vi "Insert Vi by Node.vi"(8 "error in":errorcluster caption="错误输入（无错误）", 9 "dynamic VI*":refnum<vi>, 10 "Node*":refnum<data-value>, 11 "PanelRootNode 输入":refnum<class "PanelRootNode.lvclass"> caption="DNL_LabVIEW Object in") -> (0 "error out":errorcluster caption="错误输出", 3 "PanelRootNode 输出":refnum<class "PanelRootNode.lvclass"> caption="DNL_LabVIEW Object out")   [LabVIEW 2013, in "PanelRootNode.lvclass"]
uses:
  PanelRootNode.lvclass
  PanelObject/PanelObject.lvclass
  PanelLinkNode/PanelLinkNode.lvclass/PanelLinkNode.ctl
  PanelDataNode/PanelDataNode.lvclass
  PanelLinkNode/PanelLinkNode.lvclass
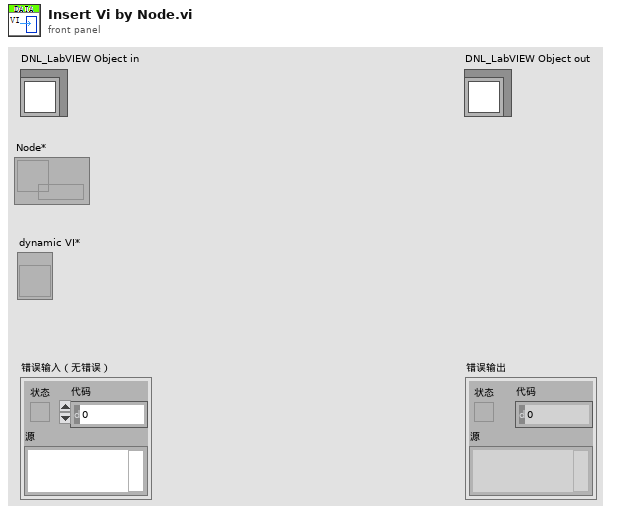
[diagram p1: front panel]
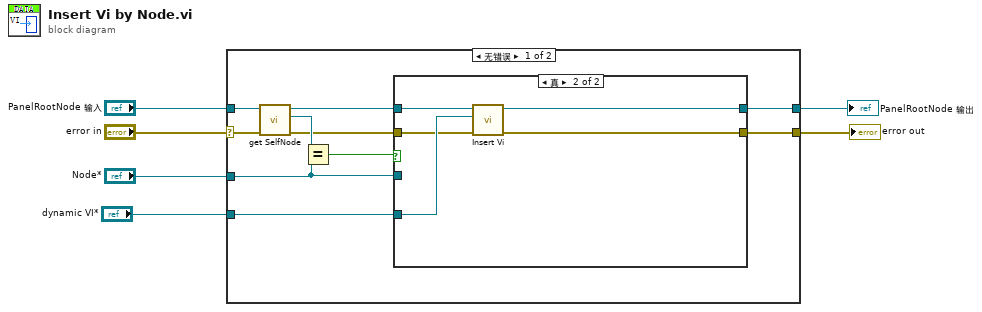
[diagram p0: block diagram]
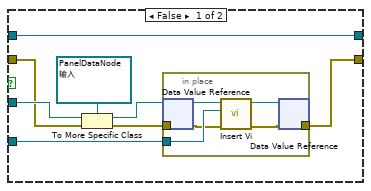
[diagram p2: hidden frame]
diagram:
  n1 = case shown="无错误" "error in" {
    selector: "error in" -> [w10 w36]
    tunnel: [w11 w36] -> w5
    tunnel: [w16 w35] -> w3
    tunnel: "PanelRootNode 输入" -> [w15 w35]
    tunnel: "Node*" -> [w13 _]
    tunnel: "dynamic VI*" -> [w8 _]
    frame No Error {
      n2 = call "get SelfNode.vi"("error in (no error)"=w10, "PanelLinkNode输入"=w15) -> ("error out"=w7:errorcluster, "SelfNode*"=w14:refnum<data-value>, "PanelLinkNode输出"=w9:refnum<class "PanelRootNode.lvclass">)  [unwired: 7 in]
      n3 = Equal?(x=w14, y=w13) -> (x = y?=w12:bool)
      n4 = case shown="真" w12 {
        tunnel: w9 -> [w17 w34]
        tunnel: w8 -> [w24 w33]
        tunnel: [w17 w32] -> w16
        tunnel: w7 -> [w19 w31]
        tunnel: w13 -> [w21 _]
        tunnel: [w23 w30] -> w11
        frame False {
          n5 = To More Specific Class(target class=refnum<data-value> refnum ("数据值引用"), reference=w21, error in=w19) -> (specific class reference=w20:refnum<data-value>, error out=w18:errorcluster)
          n6 = in-place {
            in-place-border: w24 -> [w29]
            in-place-border: w18 -> [w26]
            in-place-border: [w25] -> w23
            n7 = in-place-dvr #1(w20) -> (w28:refnum<class "PanelDataNode.lvclass">)  [unwired: 1 out]
            n8 = call-dynamic "Insert Vi.vi"("error in (no error)"=w26, "VI*"=w29, "PanelDataNode 输入"=w28) -> ("error out"=w25:errorcluster, "PanelDataNode 输出"=w27:refnum<class "PanelDataNode.lvclass">)  [unwired: 7 in]
            n9 = in-place-dvr #1(w27) -> ()  [unwired: 2 out]
          }
        }
        frame True {
          n10 = call-dynamic "Insert Vi.vi"("error in (no error)"=w31, "VI*"=w33, "PanelDataNode 输入"=w34) -> ("error out"=w30:errorcluster, "PanelDataNode 输出"=w32:refnum<class "PanelRootNode.lvclass">)  [unwired: 7 in]
        }
      }
    }
    frame Error {
    }
  }
  "error out" <- w5
  "PanelRootNode 输出" <- w3
